vi "Write Payload.vi"(8 "error in (no error)":errorcluster, 10 "Payload":u8[](array[numeric]) format="%.0x", 11 "CIF_NIChn_Fifo_U8 in":refnum<class "CIF_NIChn_Fifo_U8.lvclass">) -> (0 "error out":errorcluster, 3 "CIF_NIChn_Fifo_U8 out":refnum<class "CIF_NIChn_Fifo_U8.lvclass">)   [LabVIEW 2021, in "CIF_NIChn_Fifo_U8.lvclass"]
uses:
  CIF_NIChn_Fifo_U8.lvclass
  CIF_NIChn_Fifo_U8.lvclass/CIF_NIChn_Fifo_U8.ctl
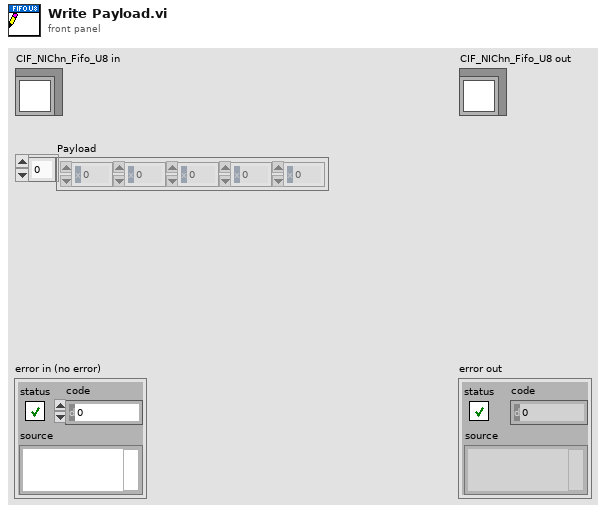
[diagram p1: front panel]
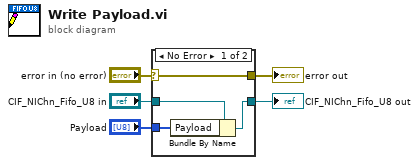
[diagram p0: block diagram]
diagram:
  n1 = case shown="No Error" "error in (no error)" {
    selector: "error in (no error)" -> [w9 w10]
    tunnel: [w9 w10] -> w4
    tunnel: [w7 w11] -> w2
    tunnel: "CIF_NIChn_Fifo_U8 in" -> [w8 w11]
    tunnel: "Payload" -> [w6 _]
    frame No Error {
      n2 = Bundle By Name(cluster=w8, "Payload"=w6) -> (w7:refnum<class "CIF_NIChn_Fifo_U8.lvclass">)
    }
    frame Error {
    }
  }
  "error out" <- w4
  "CIF_NIChn_Fifo_U8 out" <- w2
